vi "QuadratureEncoder.Measure.Digital.vi"(8 "Z":bool, 9 "B":bool, 10 "A":bool, 11 "Settings":T2={"DIRECTION"=1, "RESET VALUE"=0, "A RESET STATE"=FALSE, "B RESET STATE"=FALSE, "Z RESET STATE"=FALSE}) -> (3 "Measurement":T1)   [LabVIEW 2015, in "Speciality FPGA IO.lvlib"]
uses:
  Speciality FPGA IO.lvlib
  Types/QuadratureEncoder.Measure.Digital.Settings.ctl
  Types/QuadratureEncoder.Measure.Digital.Measurement.ctl
panel:
  out "Previous A Value":bool
  out "Previous B Value":bool
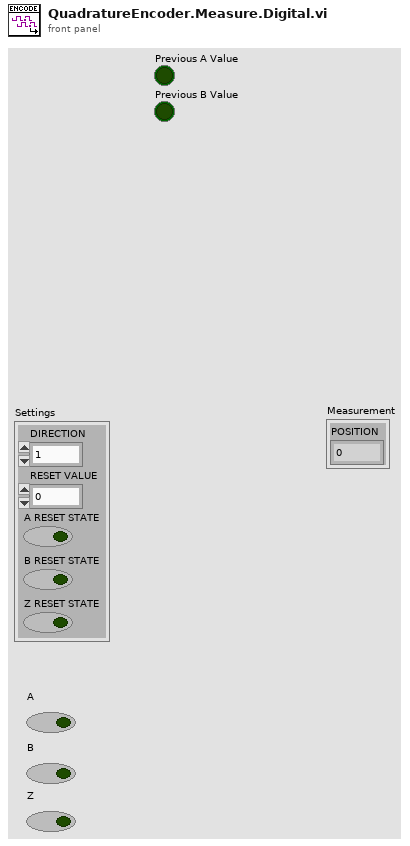
[diagram p1: front panel]
types:
  T1 = typedef "Speciality FPGA IO.lvlib/QuadratureEncoder.Measure.Digital.Measurement.ctl" = cluster{"POSITION":i32}
  T2 = typedef "Speciality FPGA IO.lvlib/QuadratureEncoder.Measure.Digital.Settings.ctl" = cluster{"DIRECTION":u8, "RESET VALUE":i32, "A RESET STATE":bool, "B RESET STATE":bool, "Z RESET STATE":bool}
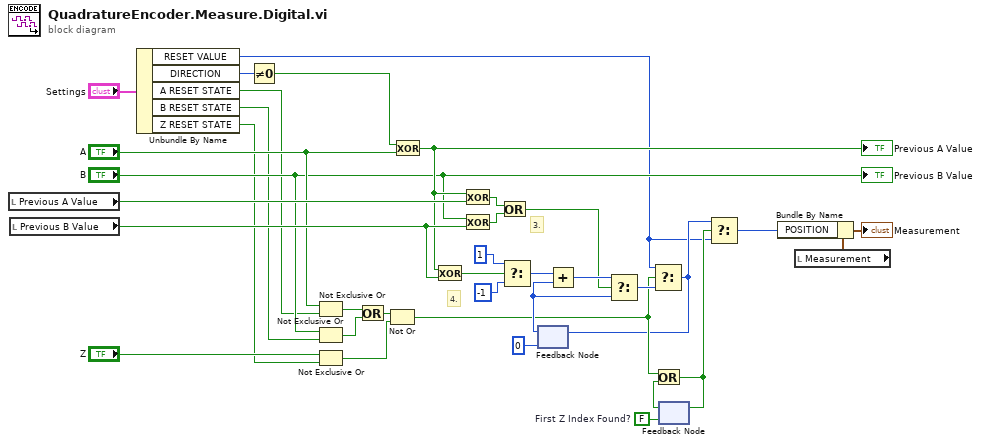
[diagram p0: block diagram]
diagram:
  w5 = FALSE  # First Z Index Found?
  # "4."
  # "3."
  n1 = local read "Previous A Value"() -> (w35:bool)
  n2 = local read "Previous B Value"() -> (w34:bool)
  n3 = Unbundle By Name("Settings") -> ("RESET VALUE"=w1:i32, "DIRECTION"=w14:u8, "A RESET STATE"=w12:bool, "B RESET STATE"=w11:bool, "Z RESET STATE"=w10:bool)
  n4 = Not Equal To 0?(x=w14) -> (x != 0?=w13:bool)
  n5 = Not Exclusive Or(1:w12, 2:"A") -> (0:w23:bool)
  n6 = Not Exclusive Or(1:w11, 2:"B") -> (0:w22:bool)
  n7 = Not Exclusive Or(1:w10, 2:"Z") -> (0:w21:bool)
  n8 = Or(x=w23, y=w22) -> (x .or. y?=w25:bool)
  n9 = Not Or(1:w21, 2:w25) -> (0:w7:bool)
  n10 = Exclusive Or(1:"A", 2:w13) -> (0:w20:bool)
  "Previous A Value" <- w20
  n11 = Exclusive Or(1:w34, 2:w20) -> (0:w26:bool)
  n12 = Exclusive Or(1:w35, 2:w20) -> (0:w28:bool)
  n13 = Exclusive Or(1:w34, 2:"B") -> (0:w29:bool)
  n14 = Or(x=w28, y=w29) -> (x .or. y?=w27:bool)
  n15 = Select(t=1, s=w26, f=-1) -> (s? t:f=w32:i32)
  n16 = feedback #1(0 ("16 bit")) -> (w16:i32)
  n17 = Add(x=w32, y=w16) -> (x+y=w33:i32)
  n18 = Select(t=w33, s=w27, f=w16) -> (s? t:f=w24:i32)
  n19 = Select(t=w1, s=w7, f=w24) -> (s? t:f=w3:i32)
  n20 = feedback-in #1(w3) -> ()
  n21 = feedback #2(w5) -> (w6:bool)
  n22 = Or(x=w7, y=w6) -> (x .or. y?=w4:bool)
  n23 = feedback-in #2(w4) -> ()
  n24 = Select(t=w3, s=w4, f=w1) -> (s? t:f=w2:i32)
  n25 = local read "Measurement"() -> (w8:T1)
  n26 = Bundle By Name(cluster=w8, "POSITION"=w2) -> (→"Measurement":T1)
  "Previous B Value" <- "B"
